vi "Send Inline Buffer.vi"(8 "error in (no error)":errorcluster, 9 "size":u64, 10 "address":u64, 11 "Plugin Interface in":refnum<class "Plugin Interface.lvclass">) -> (0 "error out":errorcluster, 3 "Plugin Interface out":refnum<class "Plugin Interface.lvclass">)   [LabVIEW 2020, in "DSF Core.lvlib" / "Plugin Interface.lvclass"]
uses:
  Plugin Interface.lvclass
  Command Parameters.ctl
  Command.ctl
  Command Data.ctl
  Send Plugin Command.vi
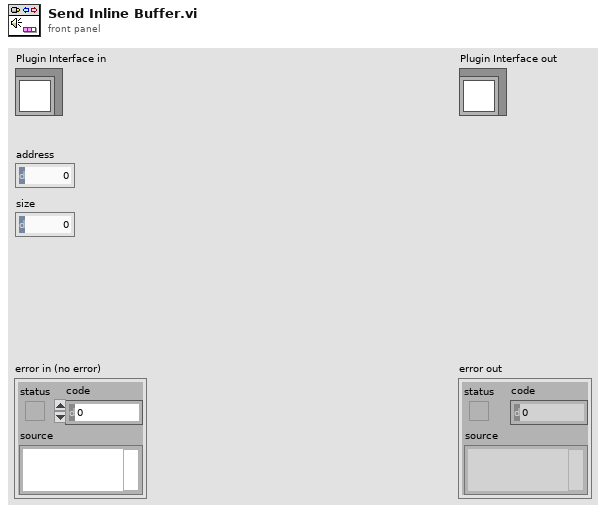
[diagram p1: front panel]
types:
  T1 = typedef "DSF Core.lvlib/Plugin Interface.lvclass/Command.ctl" = enum8{"Idle", "Start", "Set Inline Buffer", "Rx", "Tx", "Shutdown", "Error"}
  T2 = typedef "DSF Core.lvlib/Plugin Interface.lvclass/Command Parameters.ctl" = cluster{"arg1":u64, "arg2":u64}
  T3 = typedef "DSF Core.lvlib/Plugin Interface.lvclass/Command Data.ctl" = cluster{"Command":T1, "Parameters":T2}
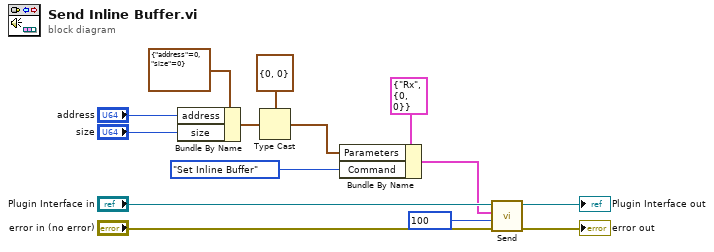
[diagram p0: block diagram]
diagram:
  n1 = Bundle By Name(cluster=cluster{"address":u64, "size":u64} {"address"=0, "size"=0}, "address"="address", "size"="size") -> (w12:cluster{"address":u64, "size":u64})
  n2 = Type Cast(type=T2 {"arg1"=0, "arg2"=0} ("Command Parameters"), x=w12) -> (*(type *) &x=w2:T2)
  n3 = Bundle By Name(cluster=T3 {"Command"=enum."Rx", "Parameters"={"arg1"=0, "arg2"=0}} ("command"), "Parameters"=w2, "Command"=Command."Set Inline Buffer") -> (w5:T3)
  n4 = call-poly "Send.vi"("error in (no error)"="error in (no error)", "timeout in ms (0)"=100, "command"=w5, "Plugin Interface in"="Plugin Interface in") -> ("error out"=→"error out":errorcluster, "Plugin Interface out"=→"Plugin Interface out":refnum<class "Plugin Interface.lvclass">)  [unwired: 6 in]
